vi "test Add-Find-Remove Remote Terminal.vi"(8 "error in":errorcluster, 11 "TestCase in":refnum<class "Scripting.lvclass">) -> (0 "error out":errorcluster, 3 "TestCase out":refnum<class "Scripting.lvclass">)   [LabVIEW 2020, in "Scripting.lvclass"]
uses:
  Scripting.lvclass
  C:/dev/git/niveristand-custom-device-testing-tools/VeriStandScriptingTestCase/VeriStandScriptingTestCase.lvclass
  <vilib>/NI VeriStand/Custom Device API/Custom Device Item Ref.ctl
  Shared/Address.ctl
  niveristand-custom-device-testing-tools/VeriStandScriptingTestCase/VeriStandScriptingTestCase.lvclass/VeriStandScriptingTestCase.ctl
  niveristand-custom-device-testing-tools/VeriStandScriptingTestCase/Read Target.vi
  NationalInstruments.VeriStand.SystemDefinitionAPI
  <vilib>/addons/_JKI Toolkits/VI Tester/TestCase.llb/TestCase.lvclass
  Scripting/AIM MIL-STD-1553 Scripting.lvlib
  <vilib>/NI VeriStand/Custom Device API/Custom Device API.lvlib
  C:/Program Files (x86)/National Instruments/LabVIEW 2020/vi.lib/addons/_JKI Toolkits/VI Tester/TestCase.llb/TestCase.lvclass
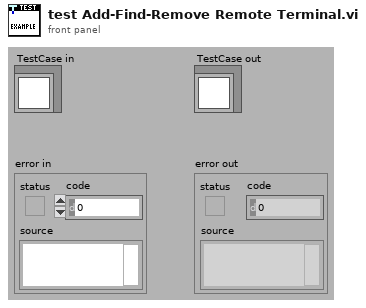
[diagram p1: front panel]
types:
  T1 = typedef "Address.ctl" = u16
  T2 = typedef "Custom Device API.lvlib/Custom Device Item Ref.ctl" = u64
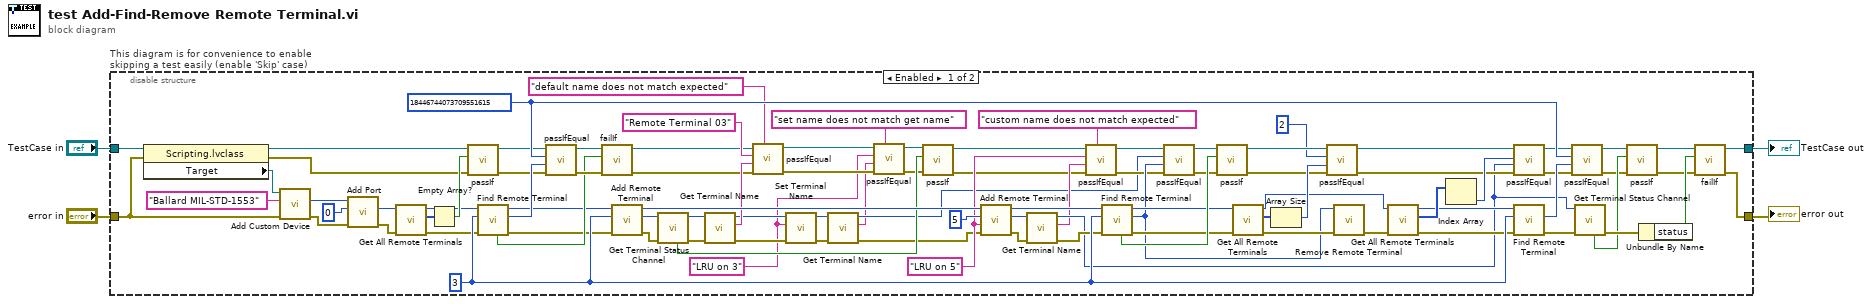
[diagram p0: block diagram]
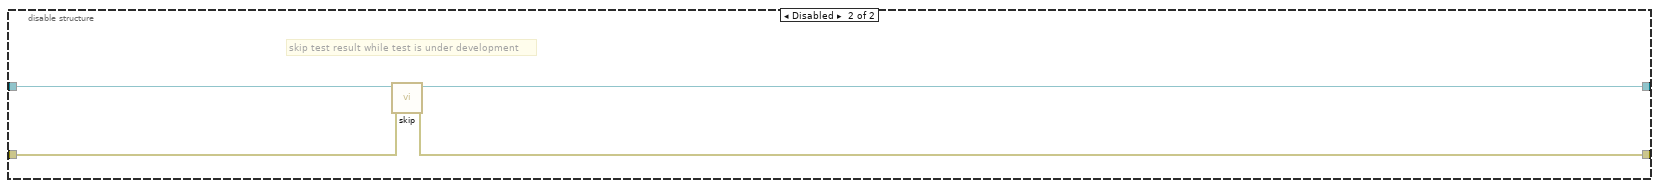
[diagram p2: hidden frame]
diagram:
  n1 = disable-structure "This diagram is for convenience to enable skipping a test easily (enable 'Skip' case)" shown="Enabled" {
    disable-tunnel: "TestCase in" -> [w98 w103]
    disable-tunnel: [w49 w101] -> w1
    disable-tunnel: [w47 w102] -> w3
    disable-tunnel: "error in" -> [w61 w100]
    frame Enabled {
      w6 = "LRU on 3" ("terminal name")
      w24 = "LRU on 5" ("terminal name")
      w86 = T1 3 ("terminal address")
      w90 = T2 18446744073709551615 ("bus controller")
      n2 = property class="Scripting.lvclass"(reference=w98, error in=w61) -> (reference out=w83:refnum<class "Scripting.lvclass">, error out=w53:errorcluster, "Target"=w97:refnum<k24>)
      n3 = call "Add Custom Device.vi"("error in"=w61, "custom device name"="Ballard MIL-STD-1553" ("name"), "target"=w97) -> ("error out"=w80:errorcluster, "custom device ref out"=w81:T2)  [unwired: 6 in, 1 out]
      n4 = call "Add Port.vi"("error in"=w80, "port number"=u16 0, "custom device ref"=w81) -> ("error out"=w79:errorcluster, "port"=w78:T2)  [unwired: 6 in, 1 out]
      n5 = call "Get All Remote Terminals.vi"("error in"=w79, "port in"=w78) -> ("error out"=w60:errorcluster, "remote terminals"=w84:T2[], "port out"=w77:T2)  [unwired: 7 in]
      n6 = Empty Array?(array=w84) -> (empty?=w85:bool)
      n7 = call-dynamic "passIf.vi"("error in (no error)"=w53, "pass"=w85, "TestCase in"=w83) -> ("error out"=w54:errorcluster, "TestCase out"=w82:refnum<class "Scripting.lvclass">)  [unwired: 7 in]
      n8 = call "Find Remote Terminal.vi"("error in"=w60, "terminal address"=w86, "port in"=w77) -> ("error out"=w59:errorcluster, "remote terminal"=w93:T2, "port out"=w67:T2, "found?"=w87:bool)  [unwired: 5 in]
      n9 = call-dynamic "passIfEqual.vi"("error in (no error)"=w54, "y"=w93, "x"=w90, "TestCase in"=w82) -> ("error out"=w94:errorcluster, "TestCase out"=w88:refnum<class "Scripting.lvclass">)  [unwired: 6 in]
      n10 = call-dynamic "failIf.vi"("error in (no error)"=w94, "fail"=w87, "TestCase in"=w88) -> ("error out"=w30:errorcluster, "TestCase out"=w31:refnum<class "Scripting.lvclass">)  [unwired: 7 in]
      n11 = call "Add Remote Terminal.vi"("error in"=w59, "terminal address"=w86, "port in"=w67) -> ("error out"=w44:errorcluster, "remote terminal"=w45:T2, "port out"=w75:T2)  [unwired: 6 in]
      n12 = call "Get Terminal Status Channel.vi"("error in"=w44, "terminal in"=w45) -> ("error out"=w34:errorcluster, "terminal out"=w35:T2, "found?"=w43:bool)  [unwired: 6 in, 1 out]
      n13 = call "Get Terminal Name.vi"("error in"=w34, "remote terminal in"=w35) -> ("error out"=w16:errorcluster, "terminal name"=w33:string, "remote terminal out"=w17:T2)  [unwired: 7 in]
      n14 = call-dynamic "passIfEqual.vi"("custom report message (\"\")"="default name does not match expected" ("custom report message (\"\")"), "error in (no error)"=w30, "y"=w33, "x"="Remote Terminal 03" ("terminal name"), "TestCase in"=w31) -> ("error out"=w14:errorcluster, "TestCase out"=w15:refnum<class "Scripting.lvclass">)  [unwired: 5 in]
      n15 = call "Set Terminal Name.vi"("error in"=w16, "terminal name"=w6, "remote terminal in"=w17) -> ("error out"=w10:errorcluster, "remote terminal out"=w11:T2)  [unwired: 7 in]
      n16 = call "Get Terminal Name.vi"("error in"=w10, "remote terminal in"=w11) -> ("error out"=w8:errorcluster, "terminal name"=w7:string, "remote terminal out"=w9:T2)  [unwired: 7 in]
      n17 = call-dynamic "passIfEqual.vi"("custom report message (\"\")"="set name does not match get name" ("custom report message (\"\")"), "error in (no error)"=w14, "y"=w7, "x"=w6, "TestCase in"=w15) -> ("error out"=w12:errorcluster, "TestCase out"=w13:refnum<class "Scripting.lvclass">)  [unwired: 5 in]
      n18 = call-dynamic "passIf.vi"("error in (no error)"=w12, "pass"=w43, "TestCase in"=w13) -> ("error out"=w22:errorcluster, "TestCase out"=w23:refnum<class "Scripting.lvclass">)  [unwired: 7 in]
      n19 = call "Add Remote Terminal.vi"("error in"=w8, "terminal name"=w24, "terminal address"=T1 5, "port in"=w75) -> ("error out"=w28:errorcluster, "remote terminal"=w29:T2, "port out"=w76:T2)  [unwired: 5 in]
      n20 = call "Get Terminal Name.vi"("error in"=w28, "remote terminal in"=w29) -> ("error out"=w27:errorcluster, "terminal name"=w25:string, "remote terminal out"=w26:T2)  [unwired: 7 in]
      n21 = call-dynamic "passIfEqual.vi"("custom report message (\"\")"="custom name does not match expected" ("custom report message (\"\")"), "error in (no error)"=w22, "y"=w25, "x"=w24, "TestCase in"=w23) -> ("error out"=w20:errorcluster, "TestCase out"=w21:refnum<class "Scripting.lvclass">)  [unwired: 5 in]
      n22 = call "Find Remote Terminal.vi"("error in"=w27, "terminal address"=w86, "port in"=w76) -> ("error out"=w58:errorcluster, "remote terminal"=w55:T2, "port out"=w74:T2, "found?"=w92:bool)  [unwired: 5 in]
      n23 = call-dynamic "passIfEqual.vi"("error in (no error)"=w20, "y"=w55, "x"=w9, "TestCase in"=w21) -> ("error out"=w91:errorcluster, "TestCase out"=w95:refnum<class "Scripting.lvclass">)  [unwired: 6 in]
      n24 = call-dynamic "passIf.vi"("error in (no error)"=w91, "pass"=w92, "TestCase in"=w95) -> ("error out"=w52:errorcluster, "TestCase out"=w73:refnum<class "Scripting.lvclass">)  [unwired: 7 in]
      n25 = call "Get All Remote Terminals.vi"("error in"=w58, "port in"=w74) -> ("error out"=w57:errorcluster, "remote terminals"=w72:T2[], "port out"=w68:T2)  [unwired: 7 in]
      n26 = Array Size(array=w72) -> (size(s)=w71:i32)
      n27 = call-dynamic "passIfEqual.vi"("error in (no error)"=w52, "y"=w71, "x"=2 ("size(s)"), "TestCase in"=w73) -> ("error out"=w51:errorcluster, "TestCase out"=w62:refnum<class "Scripting.lvclass">)  [unwired: 6 in]
      n28 = call "Remove Remote Terminal.vi"("error in"=w57, "remote terminal"=w55) -> ("error out"=w69:errorcluster)  [unwired: 9 in]
      n29 = call "Get All Remote Terminals.vi"("error in"=w69, "port in"=w68) -> ("error out"=w56:errorcluster, "remote terminals"=w66:T2[], "port out"=w63:T2)  [unwired: 7 in]
      n30 = Index Array(array=w66) -> (element=w64:T2)  [unwired: 1 in]
      n31 = call-dynamic "passIfEqual.vi"("error in (no error)"=w51, "y"=w26, "x"=w64, "TestCase in"=w62) -> ("error out"=w50:errorcluster, "TestCase out"=w65:refnum<class "Scripting.lvclass">)  [unwired: 6 in]
      n32 = call "Find Remote Terminal.vi"("error in"=w56, "terminal address"=w86, "port in"=w63) -> ("error out"=w42:errorcluster, "remote terminal"=w89:T2)  [unwired: 5 in, 2 out]
      n33 = call-dynamic "passIfEqual.vi"("error in (no error)"=w50, "y"=w89, "x"=w90, "TestCase in"=w65) -> ("error out"=w38:errorcluster, "TestCase out"=w39:refnum<class "Scripting.lvclass">)  [unwired: 6 in]
      n34 = call "Get Terminal Status Channel.vi"("error in"=w42, "terminal in"=w26) -> ("error out"=w41:errorcluster, "found?"=w40:bool)  [unwired: 6 in, 2 out]
      n35 = call-dynamic "passIf.vi"("error in (no error)"=w38, "pass"=w40, "TestCase in"=w39) -> ("error out"=w36:errorcluster, "TestCase out"=w37:refnum<class "Scripting.lvclass">)  [unwired: 7 in]
      n36 = Unbundle By Name(w41) -> ("status"=w48:bool)
      n37 = call-dynamic "failIf.vi"("error in (no error)"=w36, "fail"=w48, "TestCase in"=w37) -> ("error out"=w47:errorcluster, "TestCase out"=w49:refnum<class "Scripting.lvclass">)  [unwired: 7 in]
    }
    frame Disabled {
      # "skip test result while test is under development"
      n38 = call <vilib>:"skip.vi"("error in (no error)"=w100, "TestCase in"=w103) -> ("error out"=w102:errorcluster, "TestCase out"=w101:refnum<class "Scripting.lvclass">)  [unwired: 8 in]
    }
  }
  "error out" <- w3
  "TestCase out" <- w1
